vi "Source_ROI file columns mapping.vi"() -> (0 "ROI file columns mapping":T1)   [LabVIEW 2020]
uses:
  Typedefs/ROI file columns mapping.ctl
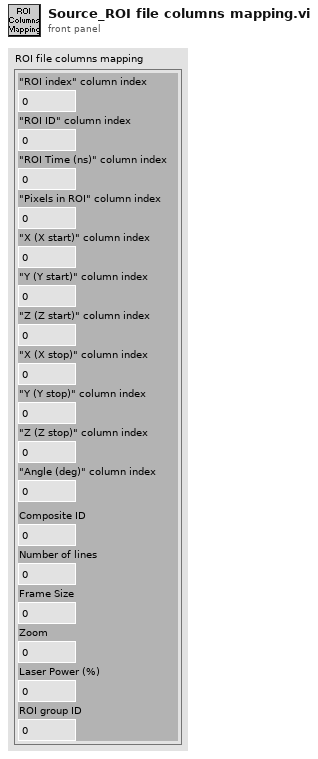
[diagram p1: front panel]
types:
  T1 = typedef "ROI file columns mapping.ctl" = cluster{"\"ROI index\" column index":i32, "\"ROI ID\" column index":i32, "\"ROI Time (ns)\" column index":i32, "\"Pixels in ROI\" column index":i32, "\"X (X start)\" column index":i32, "\"Y (Y start)\" column index":i32, "\"Z (Z start)\" column index":i32, "\"X (X stop)\" column index":i32, "\"Y (Y stop)\" column index":i32, "\"Z (Z stop)\" column index":i32, "\"Angle (deg)\" column index":i32, "Composite ID":i32, "Number of lines":i32, "Frame Size":i32, "Zoom":i32, "Laser Power (%)":i32, "ROI group ID":i32}
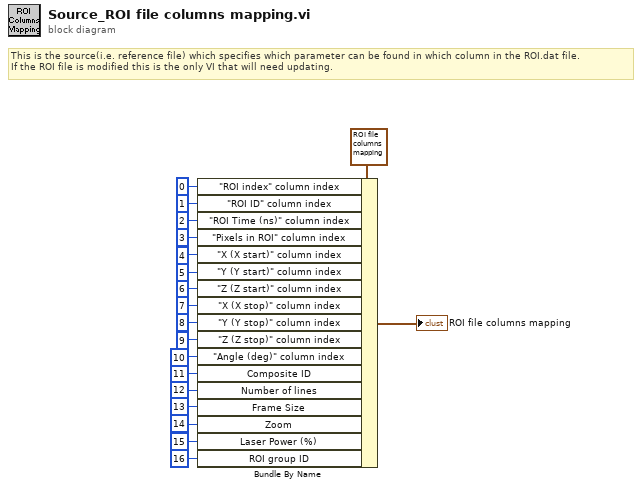
[diagram p0: block diagram]
diagram:
  # "This is the source(i.e. reference file) which specifies which parameter can be found in which column in the ROI.dat file.\nIf the ROI file is modified this is the only VI that will need updating."
  n1 = Bundle By Name(cluster=T1 {"\"ROI index\" column index"=0, "\"ROI ID\" column index"=0, "\"ROI Time (ns)\" column index"=0, "\"Pixels in ROI\" column index"=0, "\"X (X start)\" column index"=0, "\"Y (Y start)\" column index"=0, "\"Z (Z start)\" column index"=0, "\"X (X stop)\" column index"=0, "\"Y (Y stop)\" column index"=0, "\"Z (Z stop)\" column index"=0, "\"Angle (deg)\" column index"=0, "Composite ID"=0, "Number of lines"=0, "Frame Size"=0, "Zoom"=0, "Laser Power (%)"=0, "ROI group ID"=0} ("ROI file columns mapping"), "\"ROI index\" column index"=0 ("\"ROI index\" column index"), "\"ROI ID\" column index"=1 ("\"ROI ID\" column index"), "\"ROI Time (ns)\" column index"=2 ("\"ROI Time (us)\" column index"), "\"Pixels in ROI\" column index"=3 ("\"ROI Time (us)\" column index"), "\"X (X start)\" column index"=4 ("\"ROI index\" column index"), "\"Y (Y start)\" column index"=5 ("\"ROI ID\" column index"), "\"Z (Z start)\" column index"=6 ("\"ROI Time (us)\" column index"), "\"X (X stop)\" column index"=7 ("\"ROI Time (us)\" column index"), "\"Y (Y stop)\" column index"=8 ("\"ROI Time (us)\" column index"), "\"Z (Z stop)\" column index"=9 ("\"ROI index\" column index"), "\"Angle (deg)\" column index"=10 ("\"ROI ID\" column index"), "Composite ID"=11 ("\"ROI ID\" column index"), "Number of lines"=12 ("\"ROI Time (us)\" column index"), "Frame Size"=13 ("\"ROI Time (us)\" column index"), "Zoom"=14 ("\"ROI Time (us)\" column index"), "Laser Power (%)"=15 ("\"ROI index\" column index"), "ROI group ID"=16 ("\"ROI ID\" column index")) -> (→"ROI file columns mapping":T1)
